vi "Scope Measurement.vi"(0 "Scope Reference":refnum<k15>, 5 "Scope Channels":string, 7 "Shunt Resistance":dbl, 11 "error in (no error)":errorcluster, 13 "Scope Timeout (s)":dbl) -> (4 "Scope Reference Out":refnum<k15> caption="instrument handle out", 6 "Measured Output Voltage":cluster{dbl[], dbl[]}, 8 "Measured Load Current":cluster{dbl[], dbl[]}, 15 "error out":errorcluster)   [LabVIEW 2020, in "LDO Load Transient_AWG.lvlib"]
uses:
  LDO Load Transient_AWG.lvlib
  <instrlib>/niScope/Acquire/Fetch/niScope Multi Fetch Cluster.vi
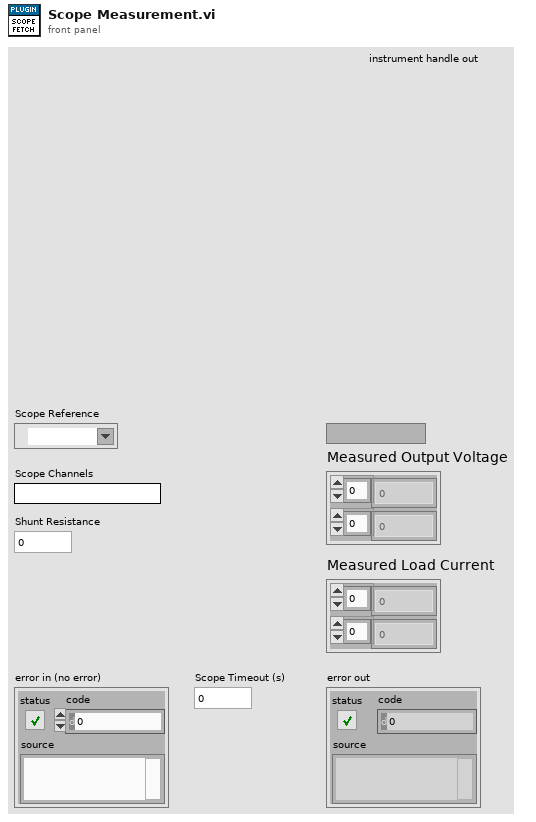
[diagram p1: front panel]
types:
  T1 = cluster{"relativeInitialX":dbl, "xIncrement":dbl, "wfm":dbl[]}[]
  T2 = cluster{"relativeInitialX":dbl, "xIncrement":dbl, "wfm":dbl[]}
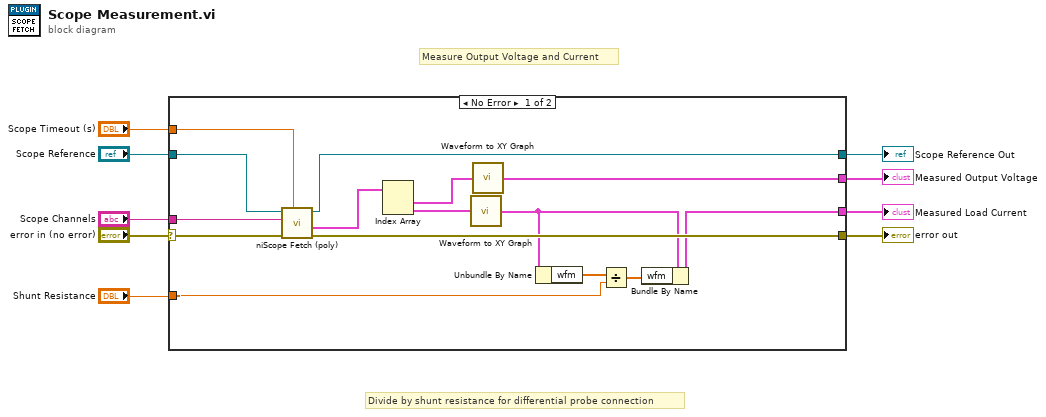
[diagram p0: block diagram]
diagram:
  # "Divide by shunt resistance for differential probe connection"
  # "Measure Output Voltage and Current"
  n1 = case shown="No Error" "error in (no error)" {
    selector: "error in (no error)" -> [w20 w26]
    tunnel: "Scope Reference" -> [w24 w25]
    tunnel: "Scope Timeout (s)" -> [w22 _]
    tunnel: [w21 w26] -> w7
    tunnel: "Scope Channels" -> [w19 _]
    tunnel: [w12 _] -> w4
    tunnel: [w17 _] -> w3
    tunnel: "Shunt Resistance" -> [w11 _]
    tunnel: [w10 w25] -> w1
    frame No Error {
      n2 = call-poly <instrlib>:"niScope Fetch (poly).vi"("timeout"=w22, "error in"=w20, "channels"=w19, "instrument handle"=w24) -> ("error out"=w21:errorcluster, "waveform"=w23:T1, "instrument handle out"=w10:refnum<k15>)  [unwired: 4 in, 1 out]
      n3 = Index Array(array=w23) -> (element #1=w16:T2, element #2=w18:T2)  [unwired: 2 in]
      n4 = call "Waveform to XY Graph.vi"("Measure Load Current"=w18) -> ("Scope Waveform"=w13:cluster{"x-axis":dbl[], "wfm":dbl[]})  [unwired: 14 in]
      n5 = call "Waveform to XY Graph.vi"("Measure Load Current"=w16) -> ("Scope Waveform"=w17:cluster{"x-axis":dbl[], "wfm":dbl[]})  [unwired: 14 in]
      n6 = Unbundle By Name(w13) -> ("wfm"=w14:dbl[])
      n7 = Divide(x=w14, y=w11) -> (x/y=w15:dbl[])
      n8 = Bundle By Name(cluster=w13, "wfm"=w15) -> (w12:cluster{"x-axis":dbl[], "wfm":dbl[]})
    }
    frame Error {
    }
  }
  "error out" <- w7
  "Measured Load Current" <- w4
  "Measured Output Voltage" <- w3
  "Scope Reference Out" <- w1
